vi "LSMcontroller_v59_PIzstage.vi"() -> ()   [LabVIEW 2015] (continued)
                                tunnel: [w4434 _] -> w4432
                                frame #0 {
                                n1728 = call "waveformparamsv2.vi"("command"="get") -> ("Params out"=w4437:T15)  [unwired: 4 in, 2 out]
                                n1729 = Unbundle By Name(w4437) -> ("DO parameters"=w4438:T18)
                                n1730 = Index Array(array=w4438, index=w4435) -> (element=w4434:T19)
                                }
                                frame #1 {
                                w4452 = 0.0 ("padding value")
                                n1731 = call "2pparameters.vi"("command"="get") -> ("params out"=w4450:T11)  [unwired: 1 in]
                                n1732 = Unbundle By Name(w4450) -> ("srate"=w4448:sgl, "Pel"=w4449:sgl)
                                n1733 = To Double Precision Float(number=w4448) -> (double precision float=w4446:dbl)
                                n1734 = To Double Precision Float(number=w4448) -> (double precision float=w4447:dbl)
                                n1735 = To Double Precision Float(number=w4449) -> (double precision float=w4442:dbl)
                                n1736 = Divide(x=1.0 ("Digital DC (%)"), y=w4442) -> (x/y=w4441:dbl)
                                n1737 = Multiply(x=100.0, y=w4441) -> (x*y=w4440:dbl)
                                n1738 = Divide(x=w4447, y=w4442) -> (x/y=w4445:dbl)
                                n1739 = call "replace DO wf param.vi"("Digital Freq (Hz)"=w4445, "Digital DC (%)"=w4440, "Digital phase"=w4452, "Sampling frequency (Hz)"=w4446, "Digital time offset (s)"=w4452, "index of DO wave"=w4444, "padding value"=w4452, "matlab wave file"=path "LT" ("matlab wave number")) -> ()  [unwired: 3 in]
                                }
                                }
                                }
                                }
                                n1740 = Build Array(w4428) -> (w4427:T18)
                                }
                                }
                                }
                                frame #9 {
                                n1741 = Build Array(w4457, w4456) -> (w4459:bool[])
                                n1742 = Boolean Array To Number(Boolean array=w4459) -> (number=w4458:u32)
                                n1743 = case shown="0" w4458 {
                                tunnel: w4455 -> [_ w4511 _ w4515]
                                tunnel: [_ w4506 _ w4512] -> w4454
                                frame 1 {
                                n1744 = call "2pparameters.vi"("command"="get") -> ("params out"=w4466:T11)  [unwired: 1 in]
                                n1745 = Unbundle By Name(w4466) -> ("wavdet"=w4467:bool, "Pel"=w4469:sgl, "refwfsize"=w4470:dbl, "Pel"=w4468:sgl)
                                n1746 = call "waveformsDObuffer.vi"("command"="get") -> ("DO wf out"=w4462:digitalwaveform[])  [unwired: 1 in]
                                n1747 = case shown="True" w4467 {
                                tunnel: [w4474 w4487] -> w4464
                                tunnel: w4468 -> [w4483 w4502]
                                tunnel: w4469 -> [w4473 w4493]
                                tunnel: w4470 -> [_ w4499]
                                frame False {
                                w4477 = u16 0 items=["unsigned binary", "offset binary", "2's complement"] ("data format (offset binary)")
                                n1748 = Initialize Array(sgl 0.0, w4473) -> (w4480:sgl[])
                                n1749 = Replace Array Subset(array=w4480, new element=sgl 1.0, index=0) -> (w4478:sgl[])
                                n1750 = Reciprocal(x=w4483) -> (1/x=w4484:sgl)
                                n1751 = Bundle By Name("Y"=w4478, "dt"=w4484) -> (w4475:waveform(sgl))  [unwired: 1 in]
                                n1752 = call-poly <vilib>:"Analog to Digital.vi"("data format (offset binary)"=w4477, "compress digital (T)"=TRUE, "full-scale range (pk-pk)"=1.0, "resolution (16 bit)"=1, "analog waveform"=w4475) -> ("digital waveform"=w4474:digitalwaveform)  [unwired: 3 in, 3 out]
                                }
                                frame True {
                                w4490 = u16 0 items=["unsigned binary", "offset binary", "2's complement"] ("data format (offset binary)")
                                n1753 = To Double Precision Float(number=w4493) -> (double precision float=w4500:dbl)
                                n1754 = Initialize Array(sgl 0.0, w4493) -> (w4495:sgl[])
                                n1755 = Divide(x=w4499, y=w4500) -> (x/y=w4497:dbl)
                                n1756 = Round Toward +Infinity(x=w4497) -> (ceil(x): smallest int >= x=w4498:dbl)
                                n1757 = Replace Array Subset(array=w4495, new element=sgl 1.0, index=0) -> (w4492:sgl[])
                                n1758 = for {
                                N: w4498 -> [_]
                                tunnel: w4492 -> [w4504]
                                tunnel: [w4504] -> w4501 mode=concatenating
                                }
                                n1759 = Reciprocal(x=w4502) -> (1/x=w4503:sgl)
                                n1760 = Bundle By Name("Y"=w4501, "dt"=w4503) -> (w4488:waveform(sgl))  [unwired: 1 in]
                                n1761 = call-poly <vilib>:"Analog to Digital.vi"("data format (offset binary)"=w4490, "compress digital (T)"=TRUE, "full-scale range (pk-pk)"=1.0, "resolution (16 bit)"=1, "analog waveform"=w4488) -> ("digital waveform"=w4487:digitalwaveform)  [unwired: 3 in, 3 out]
                                }
                                }
                                n1762 = Build Array (concatenate)(w4462, w4464) -> (w4460:digitalwaveform[])
                                n1763 = call "waveformsDObuffer.vi"("DO wf in"=w4460, "command"="set") -> ()  [unwired: 1 out]
                                }
                                frame 2 {
                                n1764 = call "waveformsDObuffer.vi"("command"="get") -> ("DO wf out"=w4508:digitalwaveform[])  [unwired: 1 in]
                                n1765 = Delete From Array(array=w4508, length=1, index=w4511) -> (deleted portion=w4506:digitalwaveform[], array with subset deleted=w4505:digitalwaveform[])
                                n1766 = call "waveformsDObuffer.vi"("DO wf in"=w4505, "command"="set") -> ()  [unwired: 1 out]
                                }
                                frame 3, Default {
                                }
                                frame 0 {
                                n1767 = local read "Measurement"() -> (w4514:T4)
                                n1768 = To Unsigned Long Integer(number=w4514) -> (unsigned 32bit integer=w4513:u32)
                                n1769 = case shown="5..7" w4513 {
                                tunnel: w4515 -> [_ w4518]
                                tunnel: [_ w4517] -> w4512
                                frame 0..4, Default {
                                }
                                frame 5..7 {
                                n1770 = call "2pparameters.vi"("command"="get") -> ("params out"=w4525:T11)  [unwired: 1 in]
                                n1771 = Unbundle By Name(w4525) -> ("wavdet"=w4526:bool, "Pel"=w4528:sgl, "refwfsize"=w4529:dbl, "srateAODO"=w4527:sgl)
                                n1772 = call "waveformsDObuffer.vi"("command"="get") -> ("DO wf out"=w4519:digitalwaveform[])  [unwired: 1 in]
                                n1773 = Index Array(array=w4519, index=w4518) -> (element=w4520:digitalwaveform)
                                n1774 = case shown="True" w4526 {
                                tunnel: [w4533 w4546] -> w4523
                                tunnel: w4527 -> [w4542 w4561]
                                tunnel: w4528 -> [w4532 w4552]
                                tunnel: w4529 -> [_ w4558]
                                frame False {
                                w4536 = u16 0 items=["unsigned binary", "offset binary", "2's complement"] ("data format (offset binary)")
                                n1775 = Initialize Array(sgl 0.0, w4532) -> (w4539:sgl[])
                                n1776 = Replace Array Subset(array=w4539, new element=sgl 1.0, index=0) -> (w4537:sgl[])
                                n1777 = Reciprocal(x=w4542) -> (1/x=w4543:sgl)
                                n1778 = Bundle By Name("Y"=w4537, "dt"=w4543) -> (w4534:waveform(sgl))  [unwired: 1 in]
                                n1779 = call-poly <vilib>:"Analog to Digital.vi"("data format (offset binary)"=w4536, "compress digital (T)"=TRUE, "full-scale range (pk-pk)"=1.0, "resolution (16 bit)"=1, "analog waveform"=w4534) -> ("digital waveform"=w4533:digitalwaveform)  [unwired: 3 in, 3 out]
                                }
                                frame True {
                                w4549 = u16 0 items=["unsigned binary", "offset binary", "2's complement"] ("data format (offset binary)")
                                n1780 = To Double Precision Float(number=w4552) -> (double precision float=w4559:dbl)
                                n1781 = Initialize Array(sgl 0.0, w4552) -> (w4554:sgl[])
                                n1782 = Divide(x=w4558, y=w4559) -> (x/y=w4556:dbl)
                                n1783 = Round Toward +Infinity(x=w4556) -> (ceil(x): smallest int >= x=w4557:dbl)
                                n1784 = Replace Array Subset(array=w4554, new element=sgl 1.0, index=0) -> (w4551:sgl[])
                                n1785 = for {
                                N: w4557 -> [_]
                                tunnel: w4551 -> [w4563]
                                tunnel: [w4563] -> w4560 mode=concatenating
                                }
                                n1786 = Reciprocal(x=w4561) -> (1/x=w4562:sgl)
                                n1787 = Bundle By Name("Y"=w4560, "dt"=w4562) -> (w4547:waveform(sgl))  [unwired: 1 in]
                                n1788 = call-poly <vilib>:"Analog to Digital.vi"("data format (offset binary)"=w4549, "compress digital (T)"=TRUE, "full-scale range (pk-pk)"=1.0, "resolution (16 bit)"=1, "analog waveform"=w4547) -> ("digital waveform"=w4546:digitalwaveform)  [unwired: 3 in, 3 out]
                                }
                                }
                                n1789 = Build Array(w4520) -> (w4517:digitalwaveform[])
                                n1790 = Replace Array Subset(array=w4519, new element=w4523, index=w4518) -> (w4516:digitalwaveform[])
                                n1791 = call "waveformsDObuffer.vi"("DO wf in"=w4516, "command"="set") -> ()  [unwired: 1 out]
                                }
                                }
                                }
                                }
                                }
                                frame #10 {
                                n1792 = local read "Meastab"() -> (w4577:enum32{"X-Y Image", "Linescan", "Timetrace"})
                                n1793 = property on="refwf" class="Ring (strict)"() -> ("RingText.Text"=w4574:string)  [unwired: 2 in, 2 out]
                                n1794 = case shown="\"Timetrace\"" w4577 {
                                tunnel: [w4579 w4580] -> w4578
                                frame "X-Y Image", Default {
                                n1795 = local read "Sampling rate"() -> (w4579:dbl)
                                }
                                frame "Timetrace" {
                                n1796 = local read "srateAODOtt"() -> (w4580:dbl)
                                }
                                }
                                n1797 = call "waveformsAObuffer.vi"("command"="get") -> ("AO wf out"=w4567:waveform(dbl)[])  [unwired: 1 in]
                                n1798 = local read "wavdet"() -> (w4575:bool)
                                n1799 = call "waveformsDObuffer.vi"("command"="get") -> ("DO wf out"=w4571:digitalwaveform[])  [unwired: 1 in]
                                n1800 = call "correctwaveformsizetemp.vi"("new sampling frequency (Hz)"=w4578, "start"=TRUE, "reference waveforms to"=w4574, "Analog waveforms in"=w4567, "stop"=FALSE, "Digital waveforms in"=w4571) -> ("analog wf out"=w4573:waveform(dbl)[], "Digital wf out"=w4566:digitalwaveform[], "measpoints"=w4576:i32)
                                n1801 = call "waveformsDObuffer.vi"("DO wf in"=w4566, "command"="set") -> ()  [unwired: 1 out]
                                n1802 = call "waveformsAObuffer.vi"("AO wf in"=w4573, "command"="set") -> ()  [unwired: 1 out]
                                n1803 = case shown="True" w4575 {
                                tunnel: w4576 -> [_ w4583]
                                tunnel: w4566 -> [_ w4581]
                                frame False {
                                }
                                frame True {
                                n1804 = local write "# of frames"(w4583) -> ()
                                n1805 = call "GetNumCamFramesv2.vi"("Digital Waveform Graph"=w4581) -> ("Numeric"=w4582:i32)  [unwired: 10 in]
                                n1806 = local write "Total Camera Frames"(w4582) -> ()
                                }
                                }
                                }
                                }
                              }
                              frame #7 {
                                # "Disabled for conversion to 64 bit"
                                n1807 = disable-structure shown="Disabled" {
                                frame Disabled {
                                n1808 = local read "Measurement"() -> (w4585:T4)
                                n1809 = case shown="\"Lifetime (scan)\"" w4585 {
                                frame "X-Y-t movie", Default {
                                }
                                frame "Lifetime (scan)" {
                                # "total acquisition time"
                                n1810 = call "2pparameters.vi"("command"="get") -> ("params out"=w4593:T11)  [unwired: 1 in]
                                n1811 = Unbundle By Name(w4593) -> ("measpoints"=w4587:i32, "srateAODO"=w4608:sgl)
                                n1812 = Divide(x=w4587, y=w4608) -> (x/y=w4586:sgl)
                                n1813 = local read "min phot"() -> (w4603:u32)
                                n1814 = local read "expected c/s"() -> (w4604:dbl)
                                n1815 = Multiply(x=w4586, y=1000.0) -> (x*y=w4596:dbl)
                                n1816 = local read "Ch1 ZeroX"() -> (w4601:i32)
                                n1817 = local read "truncate"() -> (w4602:u32)
                                n1818 = To Long Integer(number=w4596) -> (32bit integer=w4605:i32)
                                n1819 = To Long Integer(number=w4604) -> (32bit integer=w4606:i32)
                                n1820 = local read "Number of Bins"() -> (w4597:u32)
                                n1821 = local read "Ch1 Level"() -> (w4599:i32)
                                n1822 = local read "Ch0 ZeroX"() -> (w4600:i32)
                                n1823 = local write "Acquisition time"(w4605) -> ()
                                n1824 = local read "Ch0 Level"() -> (w4598:i32)
                                n1825 = call "lifetimeparameters.vi"("command"="get") -> ("Params out"=w4591:T20)  [unwired: 1 in]
                                n1826 = Add(x=100, y=w4605) -> (x+y=w4595:i32)
                                n1827 = Bundle By Name(cluster=w4591, "acq time"=w4595, "acq rate"=w4606, "# bins"=w4597, "Ch0 Level"=w4598, "Ch1 Level"=w4599, "Ch0 ZeroX"=w4600, "Ch1 ZeroX"=w4601, "min photons"=w4603, "truncate"=w4602) -> (w4590:T20)
                                n1828 = local write "Acquisition rate"(w4606) -> ()
                                n1829 = call "lifetimeparameters.vi"("Params in"=w4590, "command"="set") -> ()  [unwired: 1 out]
                                }
                                }
                                }
                                frame Enabled {
                                }
                                }
                                n1830 = local write "64bit disabled"(TRUE ("64bit disabled")) -> ()
                              }
                              frame #8 {
                                n1831 = call "2pparameters.vi"("command"="get") -> ("params out"=w4619:T11)  [unwired: 1 in]
                                n1832 = Unbundle By Name(w4619) -> ("refreshbuffer"=w4617:i32, "srate"=w4618:sgl)
                                n1833 = local read "wavdet"() -> (w4609:bool)
                                n1834 = To Double Precision Float(number=w4618) -> (double precision float=w4621:dbl)
                                n1835 = To Double Precision Float(number=w4617) -> (double precision float=w4612:dbl)
                                n1836 = case shown="False" w4609 {
                                tunnel: [w4626 w4627] -> w4611
                                frame False {
                                w4626 = 10123 items=["Finite Samples"=10178, "Continuous Samples"=10123, "Hardware Timed Single Point"=12522] ("sample mode")
                                }
                                frame True {
                                w4627 = 10123 items=["Finite Samples"=10178, "Continuous Samples"=10123, "Hardware Timed Single Point"=12522] ("sample mode")
                                }
                                }
                                n1837 = Divide(x=w4612, y=w4621) -> (x/y=w4625:dbl)
                                n1838 = Multiply(x=w4625, y=2.0) -> (x*y=w4622:dbl)
                                n1839 = Max & Min(x=w4622, y=10.0) -> (max(x,y)=w4613:dbl)  [unwired: 1 out]
                                n1840 = call "2pparameters.vi"("command"="get") -> ("params out"=w4616:T11)  [unwired: 1 in]
                                n1841 = Bundle By Name(cluster=w4616, "timeout"=w4613, "sample mode"=w4611) -> (w4614:T11)
                                n1842 = call "2pparameters.vi"("Params in"=w4614, "command"="set") -> ()  [unwired: 1 out]
                              }
                            }
                          }
                          frame #1 {
                            # "Disabled for conversion to 64 bit"
                            n1843 = call "prepAO_img.vi"() -> ("Terminal Name with Device Prefix"=w4629:tag)
                            n1844 = call "prepDO_img.vi"() -> ()  [unwired: 2 in]
                            n1845 = call "prepAI_img.vi"("triggersource"=w4629) -> ()  [unwired: 2 in]
                            n1846 = call "prepCI_img.vi"("ArmStart.DigEdge.Src"=w4629) -> ()  [unwired: 1 in]
                            n1847 = disable-structure shown="Disabled" {
                              frame Disabled {
                                n1848 = local read "Measurement"() -> (w4630:T4)
                                n1849 = case shown="\"Lifetime (contour)\"" w4630 {
                                frame "X-Y-t movie", Default {
                                }
                                frame "Lifetime (contour)" {
                                n1850 = stacked-sequence {
                                frame #0 {
                                n1851 = call "PH-temp.vi"("String"="clear" ("command")) -> ()  [unwired: 2 in, 2 out]
                                n1852 = call "PH-temp-raw.vi"("command"="empty") -> ()  [unwired: 1 in, 1 out]
                                }
                                frame #1 {
                                n1853 = call "calib.vi"() -> ()  [unwired: 1 in]
                                }
                                frame #2 {
                                n1854 = call "setup.vi"() -> ()  [unwired: 1 in]
                                }
                                }
                                }
                                }
                              }
                              frame Enabled {
                              }
                            }
                            n1855 = local write "64bit disabled"(TRUE ("64bit disabled")) -> ()
                          }
                          frame #2 {
                            n1856 = local read "save\ndata"() -> (w4633:bool)
                            n1857 = case shown="True" w4633 {
                              tunnel: w4634 -> [_ w4638]
                              frame False {
                              }
                              frame True {
                                n1858 = local read "filename prefix"() -> (w4636:string)
                                n1859 = local read "data dir"() -> (w4637:path)
                                n1860 = call "preparebinaryfiles.vi"("filename prefix"=w4636, "data dir"=w4637, "timestamp"=w4638) -> ("full-filename"=w4635:string)  [unwired: 1 in]
                                n1861 = local write "full-filename"(w4635) -> ()
                              }
                            }
                            n1862 = call "preptempbuffers_tt.vi"() -> ()  [unwired: 12 in]
                          }
                          frame #3 {
                            n1863 = local read "wavdet"() -> (w4639:bool)
                            n1864 = case shown="False" w4639 {
                              frame False {
                                n1865 = disable-structure shown="Disabled" {
                                frame Disabled {
                                n1866 = call "2pparameters.vi"("command"="get") -> ("params out"=w4641:T11)  [unwired: 1 in]
                                n1867 = Unbundle By Name(w4641) -> ("autoshutter"=w4642:bool)
                                n1868 = case shown="True" w4642 {
                                frame False {
                                }
                                frame True {
                                n1869 = call "shuttercontrol.vi"("command"="open") -> ()  [unwired: 1 in, 1 out]
                                }
                                }
                                }
                                frame Enabled {
                                }
                                }
                              }
                              frame True {
                              }
                            }
                          }
                          frame #4 {
                            n1870 = flat-sequence {
                              frame #0 {
                                # "Disabled for conversion to 64 bit"
                                n1871 = disable-structure shown="Disabled" {
                                frame Disabled {
                                n1872 = local read "Measurement"() -> (w4645:T4)
                                n1873 = case shown="\"Lifetime (contour)\"" w4645 {
                                frame "X-Y-t movie", Default {
                                }
                                frame "Lifetime (contour)" {
                                n1874 = call "runLT_img.vi"() -> ()  [unwired: 1 in]
                                }
                                }
                                }
                                frame Enabled {
                                }
                                }
                                n1875 = local write "64bit disabled"(TRUE ("64bit disabled")) -> ()
                              }
                              frame #1 {
                                n1876 = call "runAI_img.vi"() -> ()  [unwired: 12 in]
                                n1877 = call "runCI.vi"() -> ()  [unwired: 12 in]
                                n1878 = call "runDO_img.vi"() -> ()  [unwired: 12 in]
                              }
                              frame #2 {
                                n1879 = call "runAO_img.vi"() -> ()  [unwired: 12 in]
                              }
                            }
                          }
                          frame #5 {
                            # "Disabled for conversion to 64 bit"
                            n1880 = disable-structure shown="Disabled" {
                              disable-tunnel: w4647 -> [w4648 _]
                              frame Disabled {
                                w4651 = u16 0 items=["Stream to disk", "Post process", "real time process"] ("Ring")
                                n1881 = local read "T3R Data processing"() -> (w4650:u16)
                                n1882 = Equal?(x=w4650, y=w4651) -> (x = y?=w4649:bool)
                                n1883 = local read "save\ndata"() -> (w4653:bool)
                                n1884 = local read "Measurement"() -> (w4654:T4)
                                n1885 = And(x=w4653, y=w4649) -> (x .and. y?=w4652:bool)
                                n1886 = case shown="\"Lifetime (contour)\"" w4654 {
                                tunnel: w4648 -> [_ w4658]
                                tunnel: w4652 -> [_ w4656]
                                frame "X-Y-t movie", Default {
                                }
                                frame "Lifetime (contour)" {
                                n1887 = case shown="True" w4656 {
                                selector: w4656 -> [w4659 w4664]
                                tunnel: w4658 -> [_ w4662]
                                tunnel: [path "" ("appended path") w4665] -> w4657
                                tunnel: [w4659 w4664] -> w4655
                                frame False {
                                }
                                frame True {
                                n1888 = local read "filename prefix"() -> (w4663:string)
                                n1889 = local read "data dir"() -> (w4666:path)
                                n1890 = call "generatedatafilename.vi"("timestamp"=w4662, "filename prefix in"=w4663) -> ("full-filename"=w4661:string)
                                n1891 = Concatenate Strings(w4661, ".lvpt3contour" ("string")) -> (w4668:string)
                                n1892 = Build Path(base path=w4666, name or relative path=w4668) -> (appended path=w4665:path)
                                }
                                }
                                n1893 = call "collectLT_res_v1.vi"("stream?"=w4655, "data file"=w4657) -> ()  [unwired: 2 out]
                                }
                                }
                              }
                              frame Enabled {
                              }
                            }
                            n1894 = while {
                              i -> [w4671]
                              stop <- w4669 stop-if-true
                              n1895 = local read "Stop"() -> (w4679:bool)
                              n1896 = local read "Exit"() -> (w4678:bool)
                              n1897 = Increment(x=w4671) -> (x+1=w4670:i32)
                              n1898 = local write "points recorded"(w4670) -> ()
                              n1899 = Or(x=w4679, y=w4678) -> (x .or. y?=w4677:bool)
                              n1900 = case shown="False" w4677 {
                                frame False {
                                n1901 = stacked-sequence {
                                frame #0 {
                                n1902 = call "collectAI_tt_V2.vi"() -> ()  [unwired: 4 in]
                                n1903 = call "collectCI_tt.vi"() -> ("size(s)"=w4686:i32)  [unwired: 3 in]
                                n1904 = local write "scol"(w4686) -> ()
                                }
                                frame #1 {
                                n1905 = local read "Live"() -> (w4687:bool)
                                n1906 = case shown="True" w4687 {
                                frame False {
                                }
                                frame True {
                                n1907 = local read "graph1list"() -> (w4694:u16)
                                n1908 = local read "graph2list"() -> (w4693:u16)
                                n1909 = To Unsigned Word Integer(number=w4694) -> (unsigned 16bit integer=w4692:u16)
                                n1910 = To Unsigned Word Integer(number=w4693) -> (unsigned 16bit integer=w4691:u16)
                                n1911 = call "dattotrace.vi"("graph2list"=w4691, "Current Average"=sgl 1.0, "graph1list"=w4692) -> ("trace2array out"=w4689:sgl[], "trace1array out"=w4700:sgl[])
                                n1912 = local read "bin"() -> (w4701:dbl)
                                n1913 = script code="data=reshape(datain,[bin length(datain)./bin]);\ndataout=mean(data,1);\ndata2=reshape(datain2,[bin length(datain2)./bin]);\ndataout2=mean(data2,1);"("bin"=w4701, "datain"=w4700, "datain2"=w4689) -> ("dataout"=w4699:dbl[], "dataout2"=w4688:dbl[])  [unwired: 1 in, 1 out]
                                n1914 = Array Size(array=w4688) -> (size(s)=w4702:i32)
                                n1915 = Divide(x=w4702, y=2) -> (x/y=w4704:dbl)
                                n1916 = Round To Nearest(number=w4704) -> (nearest integer value=w4706:dbl)
                                n1917 = Array Size(array=w4699) -> (size(s)=w4711:i32)
                                n1918 = Delete From Array(array=w4688, length=w4706, index=0) -> (deleted portion=w4697:dbl[], array with subset deleted=w4698:dbl[])
                                n1919 = Divide(x=w4711, y=2) -> (x/y=w4709:dbl)
                                n1920 = Round To Nearest(number=w4709) -> (nearest integer value=w4707:dbl)
                                n1921 = Delete From Array(array=w4699, length=w4707, index=0) -> (deleted portion=w4696:dbl[], array with subset deleted=w4695:dbl[])
                                n1922 = local write "graph2"(w4695) -> ()
                                n1923 = local write "graph1"(w4696) -> ()
                                n1924 = local write "graph3"(w4697) -> ()
                                n1925 = local write "graph4"(w4698) -> ()
                                }
                                }
                                }
                                frame #2 {
                                n1926 = local read "save\ndata"() -> (w4712:bool)
                                n1927 = case shown="True" w4712 {
                                frame False {
                                }
                                frame True {
                                n1928 = call "savebinaryfiles.vi"() -> ()  [unwired: 1 in]
                                }
                                }
                                }
                                }
                                }
                                frame True {
                                }
                              }
                              n1929 = local read "continuous"() -> (w4674:bool)
                              n1930 = case shown="False" w4674 {
                                tunnel: w4670 -> [w4684 _]
                                tunnel: [w4683 FALSE] -> w4672
                                frame False {
                                n1931 = call "2pparameters.vi"("command"="get") -> ("params out"=w4681:T11)  [unwired: 1 in]
                                n1932 = Unbundle By Name(w4681) -> ("tt_cycles"=w4680:i32)
                                n1933 = Greater Or Equal?(x=w4684, y=w4680) -> (x >= y?=w4683:bool)
                                }
                                frame True {
                                }
                              }
                              n1934 = local read "Stop"() -> (w4676:bool)
                              n1935 = local read "Exit"() -> (w4675:bool)
                              n1936 = Or(x=w4676, y=w4675) -> (x .or. y?=w4673:bool)
                              n1937 = Or(x=w4673, y=w4672) -> (x .or. y?=w4669:bool)
                            }
                            n1938 = local write "64bit disabled"(TRUE ("64bit disabled")) -> ()
                          }
                          frame #6 {
                            # "Disabled for conversion to 64 bit"
                            n1939 = local read "Measurement"() -> (w4715:T4)
                            n1940 = disable-structure shown="Disabled" {
                              disable-tunnel: w4715 -> [w4717 _]
                              disable-tunnel: w4714 -> [w4716 _]
                              frame Disabled {
                                n1941 = case shown="\"Lifetime (contour)\"" w4717 {
                                tunnel: w4716 -> [_ w4718]
                                frame "X-Y-t movie", Default {
                                }
                                frame "Lifetime (contour)" {
                                n1942 = stacked-sequence {
                                tunnel: w4718 -> [_ w4719]
                                frame #0 {
                                n1943 = flat-sequence {
                                frame #0 {
                                n1944 = call "stoperaseLT_img.vi"() -> ()  [unwired: 1 in]
                                }
                                }
                                }
                                frame #1 {
                                w4722 = u16 0 items=["Stream to disk", "Post process", "real time process"] ("Ring")
                                n1945 = local read "T3R Data processing"() -> (w4721:u16)
                                n1946 = local read "save\ndata"() -> (w4724:bool)
                                n1947 = Equal?(x=w4721, y=w4722) -> (x = y?=w4720:bool)
                                n1948 = Not(x=w4720) -> (.not. x?=w4725:bool)
                                n1949 = And(x=w4724, y=w4725) -> (x .and. y?=w4723:bool)
                                n1950 = case shown="True" w4723 {
                                tunnel: w4719 -> [_ w4726]
                                frame False {
                                }
                                frame True {
                                n1951 = local read "filename prefix"() -> (w4727:string)
                                n1952 = local read "data dir"() -> (w4743:path)
                                n1953 = call "2pparameters.vi"("command"="get") -> ("params out"=w4738:T11)  [unwired: 1 in]
                                n1954 = call "generatedatafilename.vi"("timestamp"=w4726, "filename prefix in"=w4727) -> ("full-filename"=w4728:string)
                                n1955 = Unbundle By Name(w4738) -> ("srate"=w4736:sgl, "Pel"=w4735:sgl, "measpoints"=w4733:i32)
                                n1956 = Concatenate Strings(w4728, ".lvpt3contour" ("string")) -> (w4741:string)
                                n1957 = Build Path(base path=w4743, name or relative path=w4741) -> (appended path=w4740:path)
                                n1958 = To Unsigned Long Integer(number=w4736) -> (unsigned 32bit integer=w4737:u32)
                                n1959 = To Unsigned Long Integer(number=w4735) -> (unsigned 32bit integer=w4734:u32)
                                n1960 = To Unsigned Long Integer(number=w4733) -> (unsigned 32bit integer=w4732:u32)
                                n1961 = call "PH-temp-raw.vi"("command"="get") -> ("array out"=w4731:u32[])  [unwired: 1 in]
                                n1962 = Build Array (concatenate)(w4737, w4734, w4732, w4731) -> (w4730:u32[])
                                n1963 = Open/Create/Replace File(file path (use dialog)=w4740, operation (0:open)=T8."replace or create") -> (refnum out=w4747:refnum<file>, error out=w4746:errorcluster)  [unwired: 4 in, 1 out]
                                n1964 = Write to Binary File(file (use dialog)=w4747, data=w4730, error in=w4746, 5:FALSE ("prepend array or string size? (T)")) -> (refnum out=w4744:refnum<file>, error out=w4745:errorcluster)  [unwired: 2 in, 1 out]
                                n1965 = Close File(refnum=w4744, error in=w4745) -> ()  [unwired: 2 out]
                                }
                                }
                                }
                                }
                                }
                                }
                              }
                              frame Enabled {
                              }
                            }
                            n1966 = local write "64bit disabled"(TRUE ("64bit disabled")) -> ()
                          }
                          frame #7 {
                            n1967 = call "reset AO_DO_v3.vi"() -> ()  [unwired: 12 in]
                          }
                          frame #8 {
                            n1968 = stacked-sequence {
                              tunnel: w4763 -> [w4766 _ _ _ _ _]
                              tunnel: w4760 -> [w4765 _ _ _ _ _]
                              tunnel: w4761 -> [w4764 _ _ _ _ _]
                              tunnel: w4762 -> [_ w4815 _ _ _ _]
                              tunnel: w4758 -> [_ w4814 w4869 w4966 _ _]
                              tunnel: w4759 -> [_ w4813 w4868 w4965 _ _]
                              tunnel: w4757 -> [_ _ _ w4964 _ _]
                              tunnel: w4756 -> [_ _ _ w4963 _ _]
                              tunnel: w4755 -> [_ _ w4866 _ _ _]
                              tunnel: w4754 -> [_ _ w4865 _ _ _]
                              tunnel: w4753 -> [_ _ w4863 _ _ _]
                              tunnel: w4752 -> [_ _ w4862 _ _ _]
                              tunnel: w4751 -> [_ _ _ w4961 _ _]
                              tunnel: w4750 -> [_ _ _ w4960 _ _]
                              frame #0 {
                                n1969 = case shown="False" w4766 {
                                tunnel: w4765 -> [_ w4788]
                                tunnel: w4764 -> [_ w4787]
                                frame True {
                                n1970 = stacked-sequence {
                                seq-local: [w4767 _ _] -> [_ w4779 w4784]
                                frame #0 {
                                n1971 = call "configuration.vi"("command"="get") -> ("config out"=w4773:T12)  [unwired: 2 in, 1 out]
                                n1972 = Unbundle By Name(w4773) -> ("Voltage to Xgalvo"=w4770:i32)
                                n1973 = call "2pparameters.vi"("command"="get") -> ("params out"=w4771:T11)  [unwired: 1 in]
                                n1974 = in-place {
                                in-place-border: w4770 -> [w4778]
                                in-place-border: [w4775] -> w4767
                                n1975 = in-place-cluster #31(w4771) -> ("aAO"=w4777:u32[])
                                n1976 = call "remove channel from active arrayv2.vi"("line array in"=w4777, "line to remove"=w4778) -> ("line array out"=w4776:u32[], "index"=w4775:i32)  [unwired: 1 out]
                                n1977 = in-place-cluster #31("aAO"=w4776) -> (w4768:T11)
                                }
                                n1978 = call "2pparameters.vi"("Params in"=w4768, "command"="set") -> ()  [unwired: 1 out]
                                }
                                frame #1 {
                                n1979 = call "waveformparamsv2.vi"("command"="rem AO", "index"=w4779) -> ()  [unwired: 3 in, 3 out]
                                }
                                frame #2 {
                                n1980 = call "waveformsAObuffer.vi"("command"="get") -> ("AO wf out"=w4785:waveform(dbl)[])  [unwired: 1 in]
                                n1981 = Delete From Array(array=w4785, length=1, index=w4784) -> (array with subset deleted=w4781:waveform(dbl)[])  [unwired: 1 out]
                                n1982 = call "waveformsAObuffer.vi"("AO wf in"=w4781, "command"="set") -> ()  [unwired: 1 out]
                                }
                                }
                                }
                                frame False {
                                n1983 = stacked-sequence {
                                seq-local: [w4789 _ _] -> [_ w4797 w4808]
                                tunnel: w4788 -> [_ w4796 _]
                                tunnel: w4787 -> [_ _ w4807]
                                frame #0 {
                                n1984 = call "configuration.vi"("command"="get") -> ("config out"=w4794:T12)  [unwired: 2 in, 1 out]
                                n1985 = Unbundle By Name(w4794) -> ("Voltage to Xgalvo"=w4790:i32)
                                n1986 = call "2pparameters.vi"("command"="get") -> ("params out"=w4793:T11)  [unwired: 1 in]
                                n1987 = Unbundle By Name(w4793) -> ("aAO"=w4791:u32[])
                                n1988 = Search 1D Array(1D array=w4791, element=w4790) -> (index of element=w4789:i32)  [unwired: 1 in]
                                }
                                frame #1 {
                                n1989 = call "waveformparamsv2.vi"("command"="get") -> ("Params out"=w4800:T15)  [unwired: 4 in, 2 out]
                                n1990 = in-place {
                                in-place-border: w4797 -> [w4804]
                                in-place-border: w4796 -> [w4803]
                                n1991 = in-place-cluster #32(w4800) -> ("AO parameters"=w4805:T16)
                                n1992 = in-place {
                                in-place-border: w4803 -> [w4806]
                                n1993 = in-place-array #33(w4805, w4804) -> ()  [unwired: 1 out]
                                n1994 = in-place-array #33(w4806) -> (w4802:T16)  [unwired: 1 out]
                                }
                                n1995 = in-place-cluster #32("AO parameters"=w4802) -> (w4798:T15)
                                }
                                n1996 = call "waveformparamsv2.vi"("command"="set", "Params in"=w4798) -> ()  [unwired: 3 in, 3 out]
                                }
                                frame #2 {
                                n1997 = call "waveformsAObuffer.vi"("command"="get") -> ("AO wf out"=w4811:waveform(dbl)[])  [unwired: 1 in]
                                n1998 = Replace Array Subset(array=w4811, new element=w4807, index=w4808) -> (w4809:waveform(dbl)[])
                                n1999 = call "waveformsAObuffer.vi"("AO wf in"=w4809, "command"="set") -> ()  [unwired: 1 out]
                                }
                                }
                                }
                                }
                              }
                              frame #1 {
                                n2000 = case shown="False" w4815 {
                                tunnel: w4814 -> [_ w4837]
                                tunnel: w4813 -> [_ w4836]
                                frame True {
                                n2001 = stacked-sequence {
                                seq-local: [w4816 _ _] -> [_ w4828 w4833]
                                frame #0 {
                                n2002 = call "configuration.vi"("command"="get") -> ("config out"=w4822:T12)  [unwired: 2 in, 1 out]
                                n2003 = Unbundle By Name(w4822) -> ("Voltage to Ygalvo"=w4819:i32)
                                n2004 = call "2pparameters.vi"("command"="get") -> ("params out"=w4820:T11)  [unwired: 1 in]
                                n2005 = in-place {
                                in-place-border: w4819 -> [w4827]
                                in-place-border: [w4824] -> w4816
                                n2006 = in-place-cluster #34(w4820) -> ("aAO"=w4826:u32[])
                                n2007 = call "remove channel from active arrayv2.vi"("line array in"=w4826, "line to remove"=w4827) -> ("line array out"=w4825:u32[], "index"=w4824:i32)  [unwired: 1 out]
                                n2008 = in-place-cluster #34("aAO"=w4825) -> (w4817:T11)
                                }
                                n2009 = call "2pparameters.vi"("Params in"=w4817, "command"="set") -> ()  [unwired: 1 out]
                                }
                                frame #1 {
                                n2010 = call "waveformparamsv2.vi"("command"="rem AO", "index"=w4828) -> ()  [unwired: 3 in, 3 out]
                                }
                                frame #2 {
                                n2011 = call "waveformsAObuffer.vi"("command"="get") -> ("AO wf out"=w4834:waveform(dbl)[])  [unwired: 1 in]
                                n2012 = Delete From Array(array=w4834, length=1, index=w4833) -> (array with subset deleted=w4830:waveform(dbl)[])  [unwired: 1 out]
                                n2013 = call "waveformsAObuffer.vi"("AO wf in"=w4830, "command"="set") -> ()  [unwired: 1 out]
                                }
                                }
                                }
                                frame False {
                                n2014 = stacked-sequence {
                                seq-local: [w4838 _ _] -> [_ w4846 w4857]
                                tunnel: w4837 -> [_ w4845 _]
                                tunnel: w4836 -> [_ _ w4856]
                                frame #0 {
                                n2015 = call "configuration.vi"("command"="get") -> ("config out"=w4843:T12)  [unwired: 2 in, 1 out]
                                n2016 = Unbundle By Name(w4843) -> ("Voltage to Ygalvo"=w4839:i32)
                                n2017 = call "2pparameters.vi"("command"="get") -> ("params out"=w4842:T11)  [unwired: 1 in]
                                n2018 = Unbundle By Name(w4842) -> ("aAO"=w4840:u32[])
                                n2019 = Search 1D Array(1D array=w4840, element=w4839) -> (index of element=w4838:i32)  [unwired: 1 in]
                                }
                                frame #1 {
                                n2020 = call "waveformparamsv2.vi"("command"="get") -> ("Params out"=w4849:T15)  [unwired: 4 in, 2 out]
                                n2021 = in-place {
                                in-place-border: w4846 -> [w4853]
                                in-place-border: w4845 -> [w4852]
                                n2022 = in-place-cluster #35(w4849) -> ("AO parameters"=w4854:T16)
                                n2023 = in-place {
                                in-place-border: w4852 -> [w4855]
                                n2024 = in-place-array #36(w4854, w4853) -> ()  [unwired: 1 out]
                                n2025 = in-place-array #36(w4855) -> (w4851:T16)  [unwired: 1 out]
                                }
                                n2026 = in-place-cluster #35("AO parameters"=w4851) -> (w4847:T15)
                                }
                                n2027 = call "waveformparamsv2.vi"("command"="set", "Params in"=w4847) -> ()  [unwired: 3 in, 3 out]
                                }
                                frame #2 {
                                n2028 = call "waveformsAObuffer.vi"("command"="get") -> ("AO wf out"=w4860:waveform(dbl)[])  [unwired: 1 in]
                                n2029 = Replace Array Subset(array=w4860, new element=w4856, index=w4857) -> (w4858:waveform(dbl)[])
                                n2030 = call "waveformsAObuffer.vi"("AO wf in"=w4858, "command"="set") -> ()  [unwired: 1 out]
                                }
                                }
                                }
                                }
                              }
                              frame #2 {
                                n2031 = Build Array(w4866, w4865) -> (w4867:bool[])
                                n2032 = Boolean Array To Number(Boolean array=w4867) -> (number=w4864:u32)
                                n2033 = case shown="2" w4864 {
                                tunnel: w4869 -> [_ _ w4912]
                                tunnel: w4868 -> [_ _ w4911]
                                tunnel: w4863 -> [_ w4891 w4910]
                                tunnel: w4862 -> [_ w4890 w4909]
                                frame 1, Default {
                                n2034 = stacked-sequence {
                                seq-local: [w4870 _ _] -> [_ w4882 w4887]
                                frame #0 {
                                n2035 = call "configuration.vi"("command"="get") -> ("config out"=w4876:T12)  [unwired: 2 in, 1 out]
                                n2036 = Unbundle By Name(w4876) -> ("2P shutter"=w4873:i32)
                                n2037 = call "2pparameters.vi"("command"="get") -> ("params out"=w4874:T11)  [unwired: 1 in]
                                n2038 = in-place {
                                in-place-border: w4873 -> [w4881]
                                in-place-border: [w4878] -> w4870
                                n2039 = in-place-cluster #37(w4874) -> ("aDO"=w4880:u32[])
                                n2040 = call "remove channel from active arrayv2.vi"("line array in"=w4880, "line to remove"=w4881) -> ("line array out"=w4879:u32[], "index"=w4878:i32)  [unwired: 1 out]
                                n2041 = in-place-cluster #37("aDO"=w4879) -> (w4871:T11)
                                }
                                n2042 = call "2pparameters.vi"("Params in"=w4871, "command"="set") -> ()  [unwired: 1 out]
                                }
                                frame #1 {
                                n2043 = call "waveformparamsv2.vi"("command"="rem DO", "index"=w4882) -> ()  [unwired: 3 in, 3 out]
                                }
                                frame #2 {
                                n2044 = call "waveformsDObuffer.vi"("command"="get") -> ("DO wf out"=w4888:digitalwaveform[])  [unwired: 1 in]
                                n2045 = Delete From Array(array=w4888, length=1, index=w4887) -> (array with subset deleted=w4884:digitalwaveform[])  [unwired: 1 out]
                                n2046 = call "waveformsDObuffer.vi"("DO wf in"=w4884, "command"="set") -> ()  [unwired: 1 out]
                                }
                                }
                                }
                                frame 2 {
                                n2047 = stacked-sequence {
                                tunnel: w4891 -> [_ w4902 _]
                                tunnel: w4890 -> [_ _ w4904]
                                frame #0 {
                                n2048 = call "configuration.vi"("command"="get") -> ("config out"=w4893:T12)  [unwired: 2 in, 1 out]
                                n2049 = call "2pparameters.vi"("command"="get") -> ("params out"=w4897:T11)  [unwired: 1 in]
                                n2050 = Unbundle By Name(w4893) -> ("2P shutter"=w4892:i32)
                                n2051 = in-place {
                                in-place-border: w4892 -> [w4901]
                                n2052 = in-place-cluster #38(w4897) -> ("aDO"=w4900:u32[])
                                n2053 = call "add channel to active arrayv2.vi"("line array in"=w4900, "line to add"=w4901) -> ("line array out"=w4899:u32[])  [unwired: 2 out]
                                n2054 = in-place-cluster #38("aDO"=w4899) -> (w4895:T11)
                                }
                                n2055 = call "2pparameters.vi"("Params in"=w4895, "command"="set") -> ()  [unwired: 1 out]
                                }
                                frame #1 {
                                n2056 = call "waveformparamsv2.vi"("command"="add DO", "add DO"=w4902) -> ()  [unwired: 3 in, 3 out]
                                }
                                frame #2 {
                                n2057 = call "waveformsDObuffer.vi"("command"="get") -> ("DO wf out"=w4907:digitalwaveform[])  [unwired: 1 in]
                                n2058 = Build Array (concatenate)(w4907, w4904) -> (w4906:digitalwaveform[])
                                n2059 = call "waveformsDObuffer.vi"("DO wf in"=w4906, "command"="set") -> ()  [unwired: 1 out]
                                }
                                }
                                }
                                frame 0 {
                                n2060 = stacked-sequence {
                                seq-local: [w4913 _ _] -> [_ w4921 w4943]
                                tunnel: w4912 -> [_ _ _]
                                tunnel: w4911 -> [_ _ _]
                                tunnel: w4910 -> [_ w4920 _]
                                tunnel: w4909 -> [_ _ w4942]
                                frame #0 {
                                n2061 = call "configuration.vi"("command"="get") -> ("config out"=w4918:T12)  [unwired: 2 in, 1 out]
                                n2062 = call "2pparameters.vi"("command"="get") -> ("params out"=w4917:T11)  [unwired: 1 in]
                                n2063 = Unbundle By Name(w4918) -> ("2P shutter"=w4914:i32)
                                n2064 = Unbundle By Name(w4917) -> ("aDO"=w4915:u32[])
                                n2065 = Search 1D Array(1D array=w4915, element=w4914) -> (index of element=w4913:i32)  [unwired: 1 in]
                                }
                                frame #1 {
                                n2066 = call "2pparameters.vi"("command"="get") -> ("params out"=w4924:T11)  [unwired: 1 in]
                                n2067 = Unbundle By Name(w4924) -> ("wavdet"=w4922:bool, "autoshutter"=w4923:bool)
                                n2068 = case shown="True" w4923 {
                                tunnel: w4921 -> [_ w4928]
                                tunnel: w4922 -> [_ w4927]
                                tunnel: w4920 -> [_ w4926]
                                frame False {
                                }
                                frame True {
                                n2069 = case shown="False" w4927 {
                                tunnel: w4928 -> [w4932 _]
                                tunnel: w4926 -> [w4929 _]
                                frame False {
                                n2070 = Index Array(array=w4929, index=0) -> (element=w4930:T19)
                                n2071 = call "waveformparamsv2.vi"("command"="get") -> ("Params out"=w4935:T15)  [unwired: 4 in, 2 out]
                                n2072 = in-place {
                                in-place-border: w4932 -> [w4939]
                                in-place-border: w4930 -> [w4937]
                                n2073 = in-place-cluster #39(w4935) -> ("DO parameters"=w4940:T18)
                                n2074 = in-place {
                                in-place-border: w4937 -> [w4941]
                                n2075 = in-place-array #40(w4940, w4939) -> ()  [unwired: 1 out]
                                n2076 = in-place-array #40(w4941) -> (w4938:T18)  [unwired: 1 out]
                                }
                                n2077 = in-place-cluster #39("DO parameters"=w4938) -> (w4933:T15)
                                }
                                n2078 = call "waveformparamsv2.vi"("command"="set", "Params in"=w4933) -> ()  [unwired: 3 in, 3 out]
                                }
                                frame True {
                                }
                                }
                                }
                                }
                                }
                                frame #2 {
                                n2079 = call "2pparameters.vi"("command"="get") -> ("params out"=w4946:T11)  [unwired: 1 in]
                                n2080 = Unbundle By Name(w4946) -> ("wavdet"=w4944:bool, "autoshutter"=w4945:bool)
                                n2081 = case shown="True" w4945 {
                                tunnel: w4943 -> [_ w4950]
                                tunnel: w4944 -> [_ w4949]
                                tunnel: w4942 -> [_ w4948]
                                frame False {
                                }
                                frame True {
                                n2082 = case shown="False" w4949 {
                                tunnel: w4950 -> [w4954 _]
                                tunnel: w4948 -> [w4952 _]
                                frame False {
                                n2083 = Index Array(array=w4952, index=0) -> (element=w4951:digitalwaveform)
                                n2084 = call "waveformsDObuffer.vi"("command"="get") -> ("DO wf out"=w4956:digitalwaveform[])  [unwired: 1 in]
                                n2085 = Replace Array Subset(array=w4956, new element=w4951, index=w4954) -> (w4958:digitalwaveform[])
                                n2086 = call "waveformsDObuffer.vi"("DO wf in"=w4958, "command"="set") -> ()  [unwired: 1 out]
                                }
                                frame True {
                                }
                                }
                                }
                                }
                                }
                                }
                                }
                                }
                              }
                              frame #3 {
                                n2087 = Build Array(w4961, w4960) -> (w4962:bool[])
                                n2088 = Boolean Array To Number(Boolean array=w4962) -> (number=w4959:u32)
                                n2089 = case shown="2" w4959 {
                                tunnel: w4966 -> [_ _ w5009]
                                tunnel: w4965 -> [_ _ w5008]
                                tunnel: w4964 -> [_ w4988 w5006]
                                tunnel: w4963 -> [_ w4987 w5007]
                                frame 1, Default {
                                n2090 = stacked-sequence {
                                seq-local: [w4967 _ _] -> [_ w4979 w4984]
                                frame #0 {
                                n2091 = call "configuration.vi"("command"="get") -> ("config out"=w4973:T12)  [unwired: 2 in, 1 out]
                                n2092 = Unbundle By Name(w4973) -> ("LT timestamp"=w4970:u32)
                                n2093 = call "2pparameters.vi"("command"="get") -> ("params out"=w4971:T11)  [unwired: 1 in]
                                n2094 = in-place {
                                in-place-border: w4970 -> [w4978]
                                in-place-border: [w4975] -> w4967
                                n2095 = in-place-cluster #41(w4971) -> ("aDO"=w4977:u32[])
                                n2096 = call "remove channel from active arrayv2.vi"("line array in"=w4977, "line to remove"=w4978) -> ("line array out"=w4976:u32[], "index"=w4975:i32)  [unwired: 1 out]
                                n2097 = in-place-cluster #41("aDO"=w4976) -> (w4968:T11)
                                }
                                n2098 = call "2pparameters.vi"("Params in"=w4968, "command"="set") -> ()  [unwired: 1 out]
                                }
                                frame #1 {
                                n2099 = call "waveformparamsv2.vi"("command"="rem DO", "index"=w4979) -> ()  [unwired: 3 in, 3 out]
                                }
                                frame #2 {
                                n2100 = call "waveformsDObuffer.vi"("command"="get") -> ("DO wf out"=w4985:digitalwaveform[])  [unwired: 1 in]
                                n2101 = Delete From Array(array=w4985, length=1, index=w4984) -> (array with subset deleted=w4981:digitalwaveform[])  [unwired: 1 out]
                                n2102 = call "waveformsDObuffer.vi"("DO wf in"=w4981, "command"="set") -> ()  [unwired: 1 out]
                                }
                                }
                                }
                                frame 2 {
                                n2103 = stacked-sequence {
                                tunnel: w4988 -> [_ _ w5001]
                                tunnel: w4987 -> [_ w4999 _]
                                frame #0 {
                                n2104 = call "configuration.vi"("command"="get") -> ("config out"=w4990:T12)  [unwired: 2 in, 1 out]
                                n2105 = Unbundle By Name(w4990) -> ("LT timestamp"=w4989:u32)
                                n2106 = call "2pparameters.vi"("command"="get") -> ("params out"=w4994:T11)  [unwired: 1 in]
                                n2107 = in-place {
                                in-place-border: w4989 -> [w4998]
                                n2108 = in-place-cluster #42(w4994) -> ("aDO"=w4997:u32[])
                                n2109 = call "add channel to active arrayv2.vi"("line array in"=w4997, "line to add"=w4998) -> ("line array out"=w4996:u32[])  [unwired: 2 out]
                                n2110 = in-place-cluster #42("aDO"=w4996) -> (w4992:T11)
                                }
                                n2111 = call "2pparameters.vi"("Params in"=w4992, "command"="set") -> ()  [unwired: 1 out]
                                }
                                frame #1 {
                                n2112 = call "waveformparamsv2.vi"("command"="add DO", "add DO"=w4999) -> ()  [unwired: 3 in, 3 out]
                                }
                                frame #2 {
                                n2113 = call "waveformsDObuffer.vi"("command"="get") -> ("DO wf out"=w5004:digitalwaveform[])  [unwired: 1 in]
                                n2114 = Build Array (concatenate)(w5004, w5001) -> (w5003:digitalwaveform[])
                                n2115 = call "waveformsDObuffer.vi"("DO wf in"=w5003, "command"="set") -> ()  [unwired: 1 out]
                                }
                                }
                                }
                                frame 0 {
                                n2116 = stacked-sequence {
                                seq-local: [w5010 _ _] -> [_ w5020 w5037]
                                tunnel: w5009 -> [_ _ _]
                                tunnel: w5008 -> [_ _ _]
                                tunnel: w5007 -> [_ w5017 _]
                                tunnel: w5006 -> [_ _ w5036]
                                frame #0 {
                                n2117 = call "configuration.vi"("command"="get") -> ("config out"=w5015:T12)  [unwired: 2 in, 1 out]
                                n2118 = Unbundle By Name(w5015) -> ("LT timestamp"=w5011:u32)
                                n2119 = call "2pparameters.vi"("command"="get") -> ("params out"=w5014:T11)  [unwired: 1 in]
                                n2120 = Unbundle By Name(w5014) -> ("aDO"=w5012:u32[])
                                n2121 = Search 1D Array(1D array=w5012, element=w5011) -> (index of element=w5010:i32)  [unwired: 1 in]
                                }
                                frame #1 {
                                n2122 = local read "Measurement"() -> (w5019:T4)
                                n2123 = To Unsigned Long Integer(number=w5019) -> (unsigned 32bit integer=w5018:u32)
                                n2124 = case shown="5..7" w5018 {
                                tunnel: w5020 -> [_ w5024]
                                tunnel: w5017 -> [_ w5021]
                                frame 0..4, Default {
